vi "Convert 2D to 1D Double.vi"(11 "2D Array":dbl[][](array[numeric])) -> (1 "size(s)":i32[](array[numeric]), 3 "1D Array":dbl[](array[numeric]))   [LabVIEW 2014]
doc: "<B>Copyright</B>: (c) MHWirth 2015. All rights are reserved.\n\nThis subVI reshapes the input 1D array to 2D array based on the given sizes."
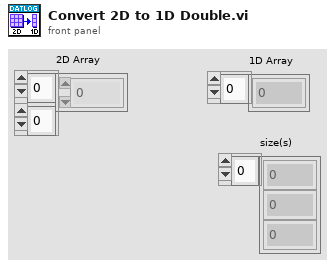
[diagram p1: front panel]
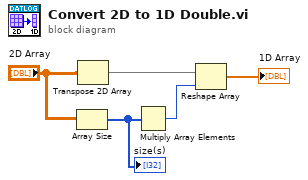
[diagram p0: block diagram]
diagram:
  n1 = Array Size(array="2D Array") -> (size(s)=w5:i32[])
  "size(s)" <- w5
  n2 = Transpose 2D Array(2D array="2D Array") -> (transposed array=w3:dbl[][])
  n3 = Multiply Array Elements(1:w5) -> (0:w2:i32)
  n4 = Reshape Array(w3, w2) -> (→"1D Array":dbl[])
